vi "GenerateData.vi"(8 "error in (no error)":errorcluster, 11 "GRMActor in":refnum<class "GeneralRMActor.lvclass">) -> (0 "error out":errorcluster, 2 "DataExchange":T1, 3 "GRMActor out":refnum<class "GeneralRMActor.lvclass">)   [LabVIEW 2020, in "GeneralRMActor.lvlib" / "GeneralRMActor.lvclass"]
uses:
  GeneralRMActor.lvclass
  Device/Device/DataExchange.ctl
  Interface/DataListener/DataListener.lvclass
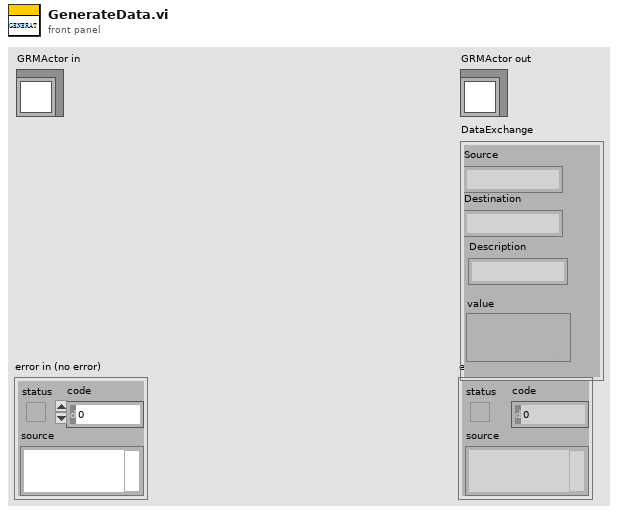
[diagram p1: front panel]
types:
  T1 = typedef "DataListener.lvclass/DataExchange.ctl" = cluster{"Source":string, "Destination":string, "Description":string, "value":variant}
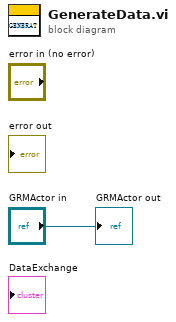
[diagram p0: block diagram]
diagram:
  "GRMActor out" <- "GRMActor in"
